vi "난수플롯이벤트.vi"() -> ()   [LabVIEW 2014]
panel:
  out "웨이브폼 차트":dbl(graph)
  in  "빈 버튼":bool
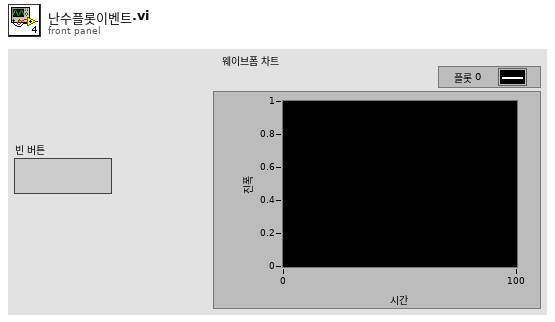
[diagram p1: front panel]
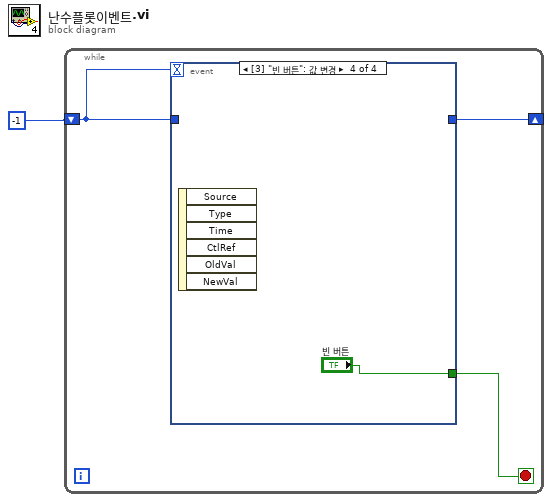
[diagram p0: block diagram]
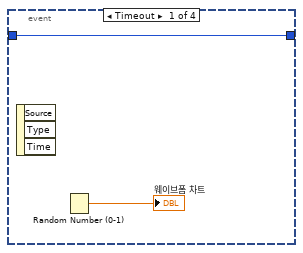
[diagram p2: hidden frame]
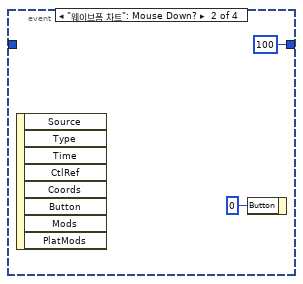
[diagram p3: hidden frame]
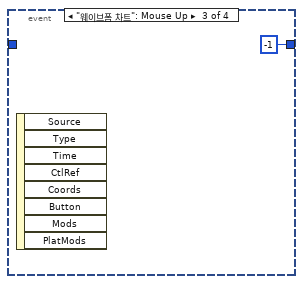
[diagram p4: hidden frame]
diagram:
  n1 = while {
    shift-right: [w3] -> _
    shift-left: -1 -> [w4]
    stop <- w2 stop-if-true
    n2 = event shown="[3] \"빈 버튼\": 값 변경" {
      selector: _ -> [_ _ _ _]
      dyn-events: _ -> [_ _ _ _]
      timeout: w4 -> [_ _ _ _]
      tunnel: w4 -> [w5 _ _ _]
      tunnel: [w5 100 -1 _] -> w3
      tunnel: [_ _ _ "빈 버튼"] -> w2
      event Timeout {
        n3 = event-data() -> ()  [unwired: 1 in, 3 out]
        n4 = Random Number (0-1)() -> (number: 0 to 1=→"웨이브폼 차트":dbl)
      }
      event "웨이브폼 차트": Mouse Down? {
        n5 = event-data() -> ()  [unwired: 1 in, 8 out]
        n6 = event-data("Button"=u16 0 ("버튼")) -> ()  [unwired: 1 in, 1 out]
      }
      event "웨이브폼 차트": Mouse Up {
        n7 = event-data() -> ()  [unwired: 1 in, 8 out]
      }
      event "빈 버튼": Value Change {
        n8 = event-data() -> ()  [unwired: 1 in, 6 out]
      }
    }
  }
